vi "XNET Read (State FlexRay Stats).vi"(0 "session in":refnum<k21>, 11 "error in (no error)":errorcluster) -> (4 "session out":refnum<k21>, 6 "FlexRay statistics":T1, 15 "error out":errorcluster)   [LabVIEW 2018]
doc: "Reads statistics for FlexRay communication using an XNET session."
uses:
  XNET FlexRay Stats.ctl
  nixlvapi.dll
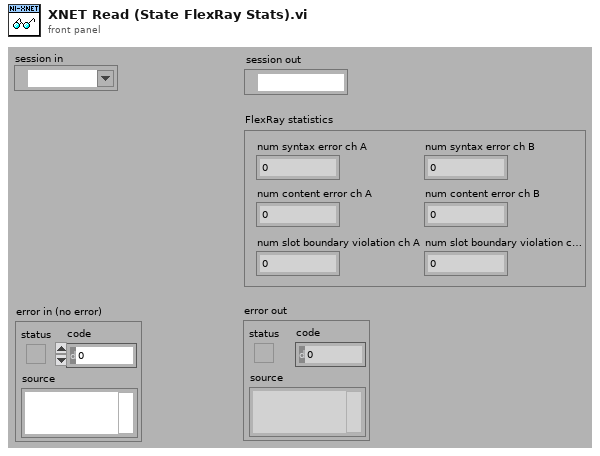
[diagram p1: front panel]
types:
  T1 = typedef "XNET FlexRay Stats.ctl" = cluster{"num syntax error ch A":u32, "num syntax error ch B":u32, "num content error ch A":u32, "num content error ch B":u32, "num slot boundary violation ch A":u32, "num slot boundary violation ch B":u32}
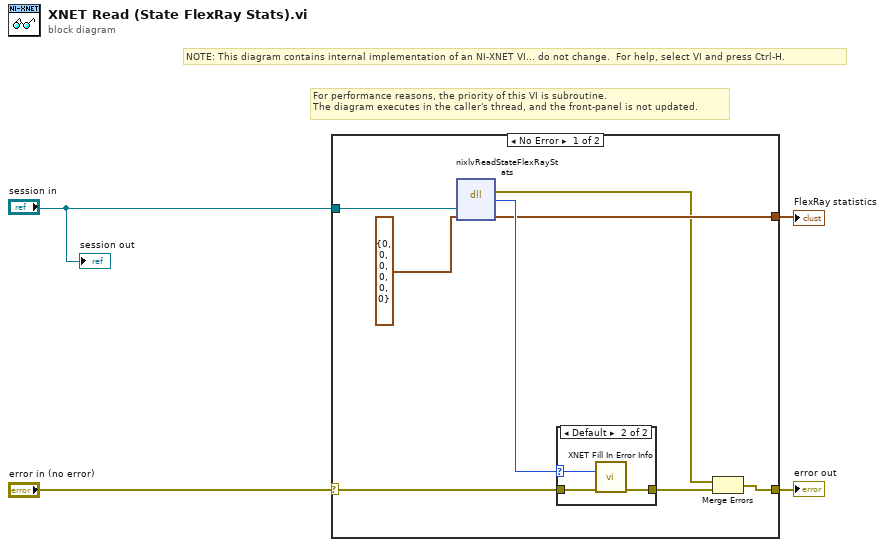
[diagram p0: block diagram]
diagram:
  # "For performance reasons, the priority of this VI is subroutine.\nThe diagram executes in the caller's thread, and the front-panel is not updated."
  # "NOTE: This diagram contains internal implementation of an NI-XNET VI... do not change.  For help, select VI and press Ctrl-H."
  n1 = case shown="No Error" "error in (no error)" {
    selector: "error in (no error)" -> [w11 w17]
    tunnel: "session in" -> [w12 _]
    tunnel: [w6 w17] -> w4
    tunnel: [w7 _] -> w1
    frame No Error {
      n2 = dll-call lib="nixlvapi.*" fn="nixlvReadStateFlexRayStats"("sessionRef"=w12, "flexRayStats"=T1 {"num syntax error ch A"=0, "num syntax error ch B"=0, "num content error ch A"=0, "num content error ch B"=0, "num slot boundary violation ch A"=0, "num slot boundary violation ch B"=0} ("FlexRay statistics")) -> (error out=w5:errorcluster, "return type"=w9:i32, "flexRayStats"=w7:T1)  [unwired: 3 in, 2 out]
      n3 = case shown="Default" w9 {
        selector: w9 -> [_ w14]
        tunnel: w11 -> [w13 w15]
        tunnel: [w13 w16] -> w10
        frame 0 {
        }
        frame Default {
          n4 = call "XNET Fill In Error Info.vi"("status code"=w14, "error in"=w15) -> ("error out"=w16:errorcluster)  [unwired: 13 out]
        }
      }
      n5 = Merge Errors(w5, w10) -> (w6:errorcluster)
    }
    frame Error {
    }
  }
  "error out" <- w4
  "FlexRay statistics" <- w1
  "session out" <- "session in"
